vi "PCUseVariant.vi"() -> ()   [LabVIEW 2014]
uses:
  MsgClusterTypedef.ctl
panel:
  in  "ButtonB":bool
  in  "ButtonA":bool
  out "NowTime":timestamp
  out "MsgString":string
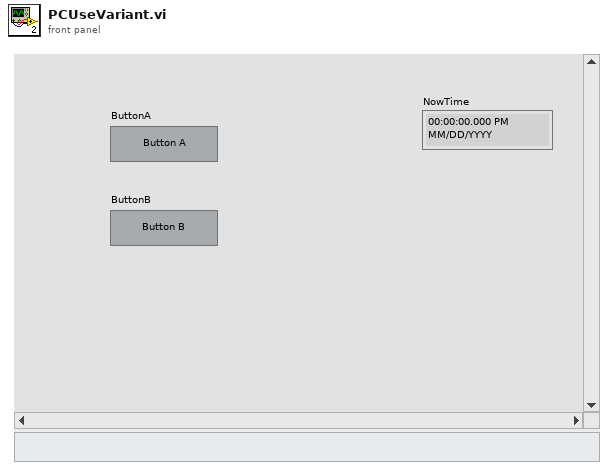
[diagram p1: front panel]
types:
  T1 = typedef "MsgClusterTypedef.ctl" = cluster{"CMD":string, "VAR":variant}
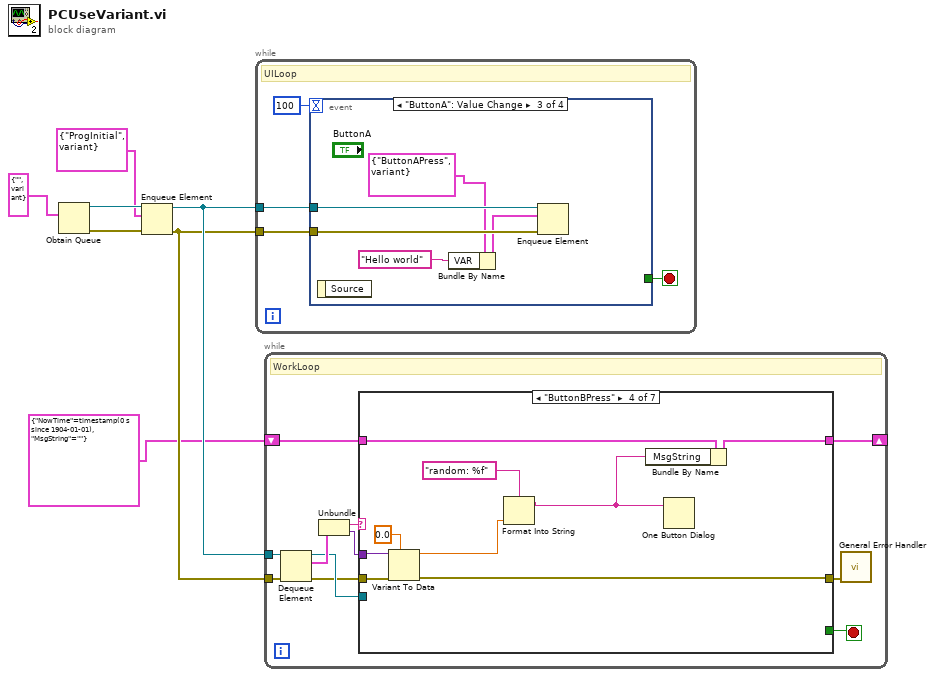
[diagram p0: block diagram]
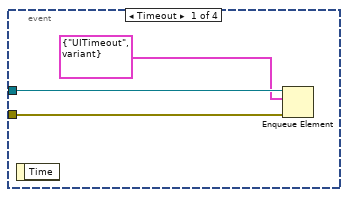
[diagram p2: hidden frame]
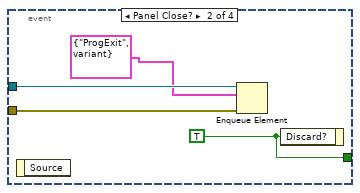
[diagram p3: hidden frame]
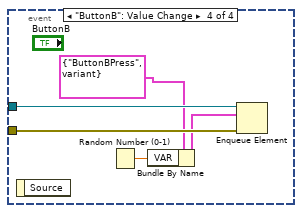
[diagram p4: hidden frame]
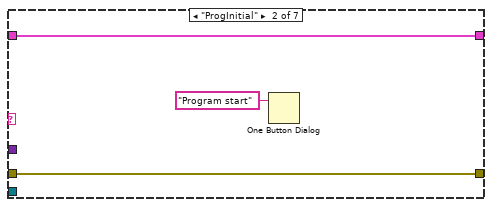
[diagram p6: hidden frame]
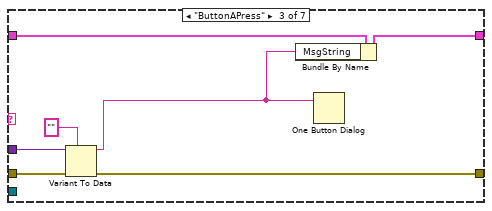
[diagram p7: hidden frame]
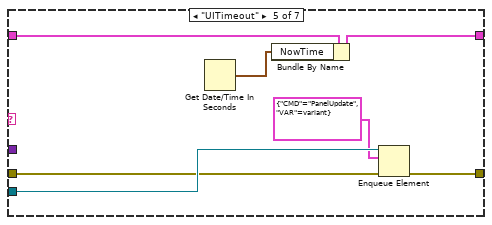
[diagram p8: hidden frame]
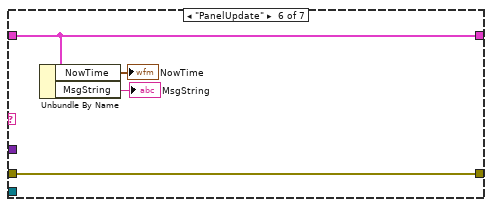
[diagram p9: hidden frame]
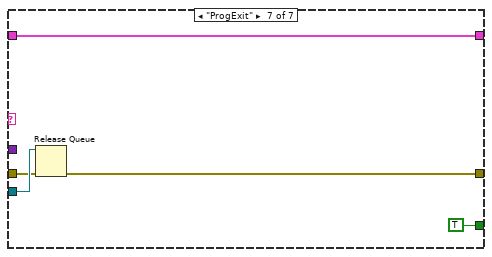
[diagram p10: hidden frame]
diagram:
  n1 = Obtain Queue(element data type=T1 {"CMD"="", "VAR"=variant}) -> (queue out=w7:refnum<queue>, error out=w6:errorcluster)  [unwired: 4 in, 1 out]
  n2 = Enqueue Element(queue=w7, element=T1 {"CMD"="ProgInitial", "VAR"=variant}, error in (no error)=w6) -> (queue out=w5:refnum<queue>, error out=w4:errorcluster)  [unwired: 1 in, 1 out]
  n3 = while {
    tunnel: w5 -> [w10]
    tunnel: w4 -> [w9]
    stop <- w8 stop-if-true
    # "UILoop"
    n4 = event shown="[2] \"ButtonA\": Value Change" {
      selector: _ -> [_ _ _ _]
      dyn-events: _ -> [_ _ _ _]
      timeout: 100 -> [_ _ _ _]
      tunnel: w10 -> [w14 w18 w23 w28]
      tunnel: w9 -> [w13 w17 w22 w27]
      tunnel: [_ w16 _ _] -> w8
      event Timeout {
        n5 = event-data() -> ()  [unwired: 1 in, 1 out]
        n6 = Enqueue Element(queue=w14, element=T1 {"CMD"="UITimeout", "VAR"=variant}, error in (no error)=w13) -> ()  [unwired: 1 in, 3 out]
      }
      event Panel Close? {
        w16 = TRUE ("Discard?")
        n7 = event-data() -> ()  [unwired: 1 in, 1 out]
        n8 = Enqueue Element(queue=w18, element=T1 {"CMD"="ProgExit", "VAR"=variant}, error in (no error)=w17) -> ()  [unwired: 1 in, 3 out]
        n9 = event-data("Discard?"=w16) -> ()  [unwired: 1 in, 1 out]
      }
      event "ButtonA": Value Change {
        n10 = event-data() -> ()  [unwired: 1 in, 1 out]
        n11 = Bundle By Name(cluster=T1 {"CMD"="ButtonAPress", "VAR"=variant}, "VAR"="Hello world") -> (w20:T1)
        n12 = Enqueue Element(queue=w23, element=w20, error in (no error)=w22) -> ()  [unwired: 1 in, 3 out]
      }
      event "ButtonB": Value Change {
        n13 = event-data() -> ()  [unwired: 1 in, 1 out]
        n14 = Random Number (0-1)() -> (number: 0 to 1=w24:dbl)
        n15 = Bundle By Name(cluster=T1 {"CMD"="ButtonBPress", "VAR"=variant}, "VAR"=w24) -> (w25:T1)
        n16 = Enqueue Element(queue=w28, element=w25, error in (no error)=w27) -> ()  [unwired: 1 in, 3 out]
      }
    }
  }
  n17 = while {
    tunnel: w5 -> [w39]
    tunnel: w4 -> [w38]
    shift-right: [w36] -> _
    shift-left: cluster{"NowTime":timestamp, "MsgString":string} {"NowTime"=timestamp(0 s since 1904-01-01), "MsgString"=""} -> [w35]
    stop <- w32 stop-if-true
    # "WorkLoop"
    n18 = Dequeue Element(queue=w39, error in (no error)=w38) -> (queue out=w34:refnum<queue>, element=w37:T1, error out=w33:errorcluster)  [unwired: 1 in, 1 out]
    n19 = Unbundle(w37) -> ("CMD"=w31:string, "VAR"=w30:variant)
    n20 = case shown="\"ButtonBPress\"" w31 {
      tunnel: [w41 w43 w50 w59 w66 w71 w76] -> w36
      tunnel: w35 -> [w41 w43 w51 w60 w67 w71 w76]
      tunnel: w34 -> [_ _ _ _ w64 _ w75]
      tunnel: w33 -> [w40 w42 w49 w58 w63 w68 w74]
      tunnel: [_ _ _ _ _ _ TRUE ("Discard?")] -> w32
      tunnel: w30 -> [_ _ w48 w57 _ _ _]
      tunnel: [w40 w42 w45 w52 w61 w68 w72] -> w29
      frame Default {
      }
      frame "ProgInitial" {
        n21 = One Button Dialog(message="Program start") -> ()  [unwired: 1 in, 1 out]
      }
      frame "ButtonAPress" {
        n22 = Variant To Data(error in=w49, type="", Variant=w48) -> (data=w46:string, error out=w45:errorcluster)
        n23 = Bundle By Name(cluster=w51, "MsgString"=w46) -> (w50:cluster{"NowTime":timestamp, "MsgString":string})
        n24 = One Button Dialog(message=w46) -> ()  [unwired: 1 in, 1 out]
      }
      frame "ButtonBPress" {
        n25 = Variant To Data(error in=w58, type=0.0, Variant=w57) -> (data=w54:dbl, error out=w52:errorcluster)
        n26 = Format Into String(format string="random: %f", w54) -> (resulting string=w53:string)  [unwired: 2 in, 1 out]
        n27 = Bundle By Name(cluster=w60, "MsgString"=w53) -> (w59:cluster{"NowTime":timestamp, "MsgString":string})
        n28 = One Button Dialog(message=w53) -> ()  [unwired: 1 in, 1 out]
      }
      frame "UITimeout" {
        n29 = Get Date/Time In Seconds() -> (seconds since 1Jan1904=w65:timestamp)
        n30 = Bundle By Name(cluster=w67, "NowTime"=w65) -> (w66:cluster{"NowTime":timestamp, "MsgString":string})
        n31 = Enqueue Element(queue=w64, element=T1 {"CMD"="PanelUpdate", "VAR"=variant}, error in (no error)=w63) -> (error out=w61:errorcluster)  [unwired: 1 in, 2 out]
      }
      frame "PanelUpdate" {
        n32 = Unbundle By Name(w71) -> ("NowTime"=→"NowTime":timestamp, "MsgString"=→"MsgString":string)
      }
      frame "ProgExit" {
        n33 = Release Queue(queue=w75, error in (no error)=w74) -> (error out=w72:errorcluster)  [unwired: 1 in, 2 out]
      }
    }
    n34 = call <vilib>:"General Error Handler.vi"("error in (no error)"=w29) -> ()  [unwired: 10 in, 5 out]
  }
